vi "Make_CRC.vi"(1 "数组输入":u8[](array[numeric]) format="%x") -> (0 "CRC_反":u16 format="%x")   [LabVIEW 2015]
doc: "数组输入：输入10个数据字节 （0-10）；\n字符串输出：把输入的10个字节经过ModBus CRC校验后生成 CRC_H,CRC_L 之后，转化成字符串 ；\n输出形式可选"
panel:
  out "CRC_正":u32 format="%x"
  out "L_CRC":u32 format="%x"
  out "H_CRC":u32 format="%x"
  out "字符串输出":string
  out "M":u8[](array[numeric])
  out "Output":u8[](array[numeric])
  out "字符串":string
  # "输入10个字节，a[0]-a[9]为数据字节，需要生成2个ModBus CRC校验字节， CRC_H 、CRC_L"
  # "输入类型：无符号数组（10个字节）"
  # "输出类型：可自选"
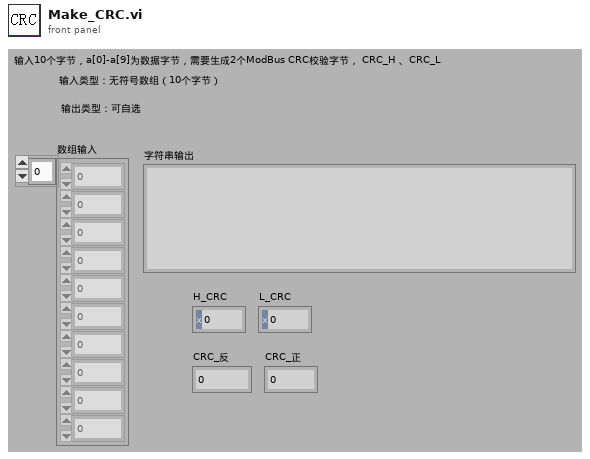
[diagram p1: front panel]
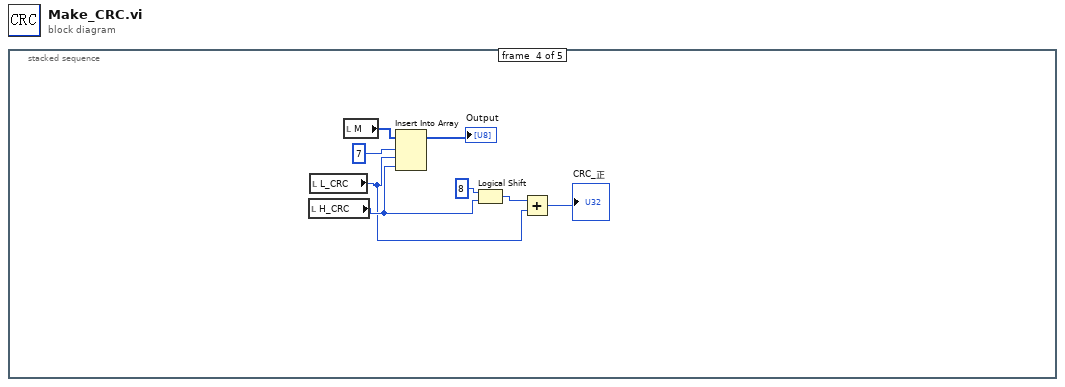
[diagram p0: block diagram]
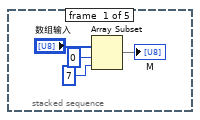
[diagram p2: hidden frame]
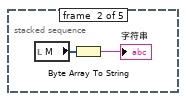
[diagram p3: hidden frame]
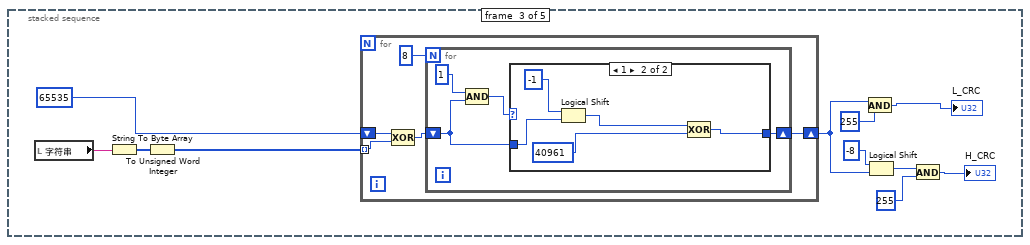
[diagram p4: hidden frame]
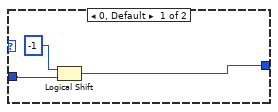
[diagram p5: hidden frame]
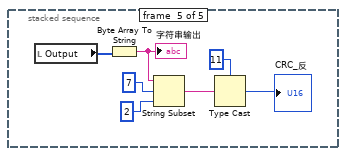
[diagram p6: hidden frame]
diagram:
  n1 = stacked-sequence {
    frame #0 {
      n2 = Array Subset(array="数组输入", index=0 ("索引"), length=7 ("索引")) -> (→"M":u8[])
    }
    frame #1 {
      n3 = local read "M"() -> (w6:u8[])
      n4 = Byte Array To String(unsigned byte array=w6) -> (string=→"字符串":string)
    }
    frame #2 {
      n5 = local read "字符串"() -> (w9:string)
      n6 = String To Byte Array(string=w9) -> (unsigned byte array=w16:u8[])
      n7 = To Unsigned Word Integer(number=w16) -> (unsigned 16bit integer=w15:u16[])
      n8 = for {
        shift-right: [w19] -> w10
        shift-left: u16 65535 -> [w20]
        tunnel: w15 -> [w18] mode=indexing
        n9 = Compound Arithmetic op=XOR(w20, w18) -> (w21:u32)
        n10 = for {
          N: 8 -> [_]
          shift-right: [w25] -> w19
          shift-left: w21 -> [w24]
          n11 = Compound Arithmetic op=AND(u16 1, w24) -> (w23:u32)
          n12 = case shown="1" w23 {
            tunnel: [w28 w33] -> w25
            tunnel: w24 -> [w27 w30]
            frame 0, Default {
              n13 = Logical Shift(y=i16 -1, x=w27) -> (x << y=w28:u32)
            }
            frame 1 {
              n14 = Logical Shift(y=i16 -1, x=w30) -> (x << y=w32:u32)
              n15 = Compound Arithmetic op=XOR(w32, u32 40961) -> (w33:u32)
            }
          }
        }
      }
      n16 = And(x=w10, y=u16 255) -> (x .and. y?=→"L_CRC":u32)
      n17 = Logical Shift(y=i16 -8, x=w10) -> (x << y=w12:u32)
      n18 = And(x=w12, y=u16 255) -> (x .and. y?=→"H_CRC":u32)
    }
    frame #3 {
      n19 = local read "H_CRC"() -> (w38:u32)
      n20 = local read "L_CRC"() -> (w36:u32)
      n21 = local read "M"() -> (w40:u8[])
      n22 = Insert Into Array(array=w40, index=7, new element #1=w36, new element #2=w38) -> (→"Output":u8[])
      n23 = Logical Shift(y=8, x=w38) -> (x << y=w37:u32)
      n24 = Add(x=w37, y=w36) -> (x+y=→"CRC_正":u32)
    }
    frame #4 {
      n25 = local read "Output"() -> (w49:u8[])
      n26 = Byte Array To String(unsigned byte array=w49) -> (string=w48:string)
      "字符串输出" <- w48
      n27 = String Subset(string=w48, offset (0)=7, length (rest)=2) -> (substring=w44:string)
      n28 = Type Cast(type=u16 11, x=w44) -> (*(type *) &x=→"CRC_反":u16)
    }
  }
